vi "Query RF Switch Matrix.vi"(10 "Basic Path":path) -> (1 "Path":path, 3 "Matrix List":string[](array[string]))   [LabVIEW 2011]
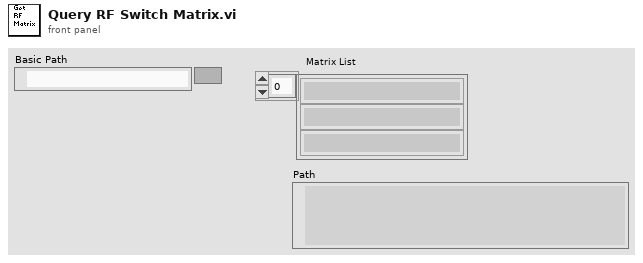
[diagram p1: front panel]
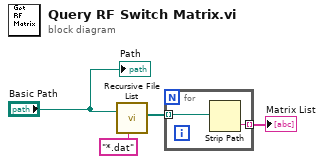
[diagram p0: block diagram]
diagram:
  n1 = call <vilib>:"Recursive File List.vi"("pattern"="*.dat", "Folder Path"="Basic Path") -> ("All Files in Dir"=w3:path[])  [unwired: 5 in, 4 out]
  n2 = for {
    tunnel: w3 -> [w6] mode=indexing
    tunnel: [w5] -> w4 mode=indexing
    n3 = Strip Path(path=w6) -> (name=w5:string)  [unwired: 1 out]
  }
  "Matrix List" <- w4
  "Path" <- "Basic Path"
